vi "telemetryHardpointData.vi"(8 "error in (no error)":errorcluster, 11 "Publisher in":refnum<class "Publisher.lvclass">) -> (0 "error out":errorcluster, 3 "Publisher out":refnum<class "Publisher.lvclass">)   [LabVIEW 2016, in "Publisher.lvclass"]
uses:
  Publisher.lvclass
  Publisher.lvclass/Publisher.ctl
  Communicator/Communicator/Communicator.lvclass
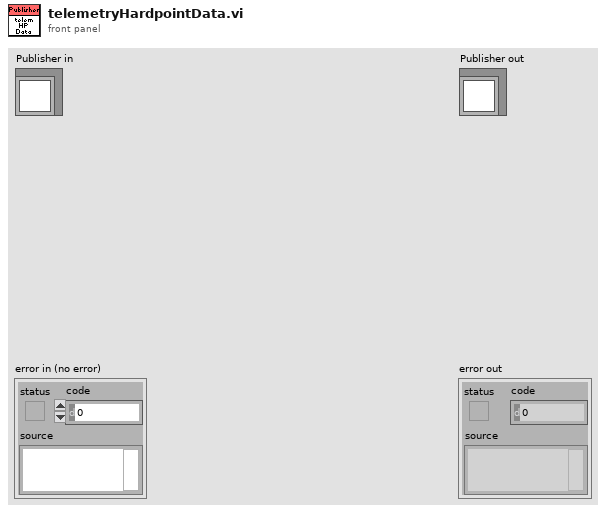
[diagram p1: front panel]
types:
  T1 = typedef "M1M3SupportTopics.lvlib/TelemetryHardpointData.ctl" = cluster{"Timestamp":T2, "StepsCommanded":i16[], "Force":sgl[], "Encoder":i32[], "ILCFault":bool[], "CWLimitOperated":bool[], "CCWLimitOperated":bool[], "BroadcastCounter":u8[]}
  T2 = typedef "M1M3SupportTopics.lvlib/Timestamp.ctl" = dbl
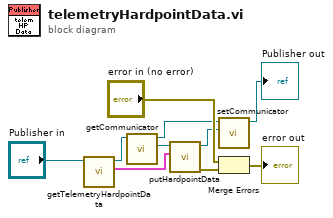
[diagram p0: block diagram]
diagram:
  n1 = call "getTelemetryHardpointData.vi"("Publisher in"="Publisher in") -> ("TelemetryHardpointData"=w7:T1, "Publisher out"=w2:refnum<class "Publisher.lvclass">)  [unwired: 9 in]
  n2 = call "getCommunicator.vi"("Publisher in"=w2) -> ("Communicator"=w6:refnum<class "Communicator.lvclass">, "Publisher out"=w3:refnum<class "Publisher.lvclass">)  [unwired: 9 in]
  n3 = call-dynamic "putHardpointData.vi"("TelemetryHardpointData"=w7, "Communicator in"=w6) -> ("error out"=w4:errorcluster, "Communicator out"=w5:refnum<class "Communicator.lvclass">)  [unwired: 8 in]
  n4 = call "setCommunicator.vi"("Communicator"=w5, "Publisher in"=w3) -> ("Publisher out"=→"Publisher out":refnum<class "Publisher.lvclass">)  [unwired: 9 in]
  n5 = Merge Errors("error in (no error)", w4) -> (→"error out":errorcluster)
